vi "Main_Motor_Evaluation_Force.vi"(0 "VISA Refnum in":refnum<visa-resource-name>, 5 "Positions to reach":dbl[](array[numeric]), 11 "error in (no error)":errorcluster) -> (4 "VISA Refnum out":refnum<visa-resource-name>, 6 "Actual positions":dbl[](array[numeric]), 8 "Current (mA)":dbl[](array[numeric]), 15 "error out":errorcluster)   [LabVIEW 2015]
uses:
  <instrlib>/Dynamixel Motor/Dynamixel Motor.lvlib
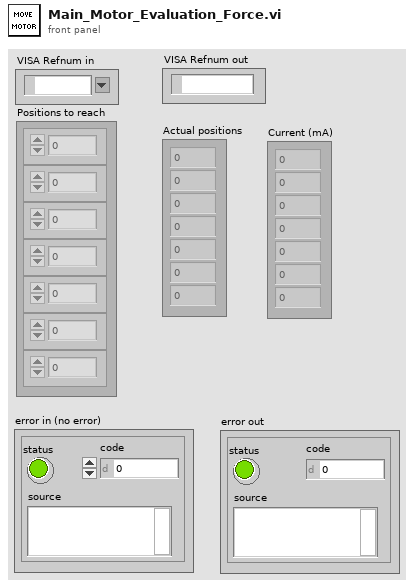
[diagram p1: front panel]
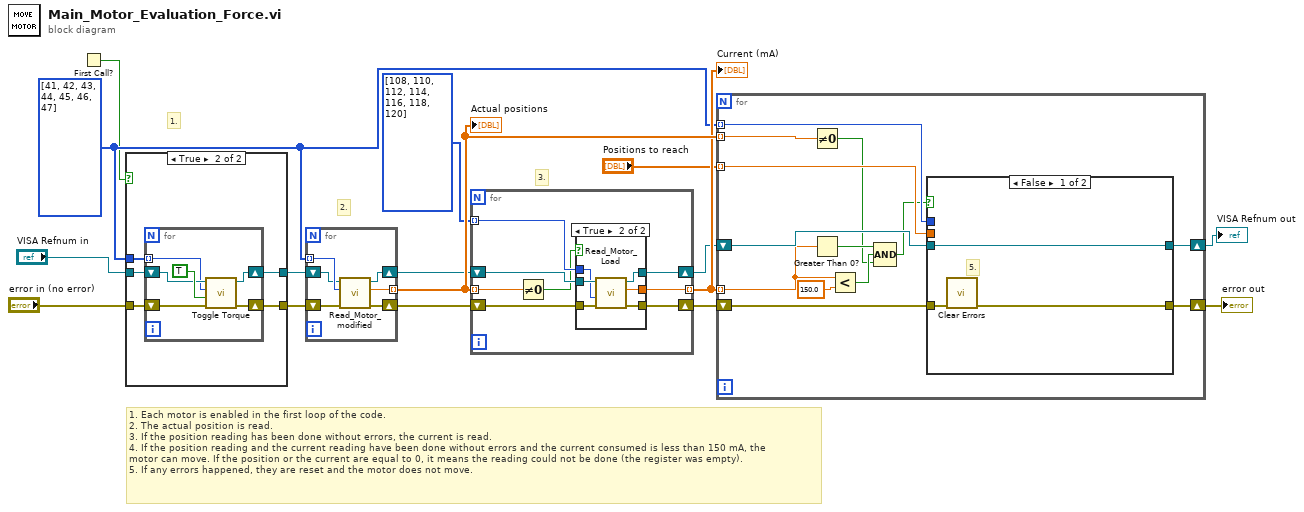
[diagram p0: block diagram]
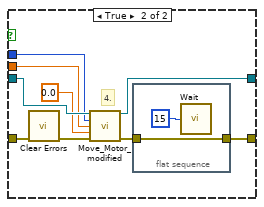
[diagram p2: hidden frame]
diagram:
  w6 = i32[] [41, 42, 43, 44, 45, 46, 47] ("y")
  # "3."
  # "2."
  # "1."
  # "1. Each motor is enabled in the first loop of the code.\n2. The actual position is read.\n3. If the position reading has been done without errors, the current is read.\n4. If the position reading and the current reading have been done without errors and the current consumed is less than 150 mA, the \nmotor can move. If the position or the current are equal to 0, it means the reading could not be done (the register was empty).\n5. If any errors happened, they are reset and the motor does not move."
  n1 = First Call?() -> (First Call?: T/F=w5:bool)
  n2 = case shown="True" w5 {
    tunnel: "VISA Refnum in" -> [w17 w23]
    tunnel: "error in (no error)" -> [w18 w22]
    tunnel: [w17 w21] -> w9
    tunnel: [w18 w20] -> w10
    tunnel: w6 -> [_ w19]
    frame False {
    }
    frame True {
      n3 = for {
        shift-right: [w27] -> w21
        shift-left: w23 -> [w28]
        shift-right: [w25] -> w20
        shift-left: w22 -> [w26]
        tunnel: w19 -> [w24] mode=indexing
        n4 = call <instrlib>:"Toggle Torque.vi"("error in (no error)"=w26, "Toggle torque (OFF)"=TRUE, "Motor ID (0)"=w24, "VISA resource name"=w28) -> ("error out"=w25:errorcluster, "VISA resource name out"=w27:refnum<visa-resource-name>)  [unwired: 6 in]
      }
    }
  }
  n5 = for {
    tunnel: w6 -> [w35] mode=indexing
    shift-right: [w30] -> w12
    shift-left: w10 -> [w34]
    shift-right: [w32] -> w11
    shift-left: w9 -> [w33]
    tunnel: [w31] -> w16 mode=indexing
    n6 = call "Read_Motor_modified.vi"("error in (no error)"=w34, "Motor ID (0)"=w35, "VISA Refnum in"=w33) -> ("error out"=w30:errorcluster, "Position"=w31:dbl, "VISA Refnum out"=w32:refnum<visa-resource-name>)  [unwired: 6 in]
  }
  "Actual positions" <- w16
  n7 = for {
    shift-right: [w42] -> w13
    shift-left: w11 -> [w43]
    shift-right: [w39] -> w14
    shift-left: w12 -> [w41]
    tunnel: [w38] -> w15 mode=indexing
    tunnel: u8[] [108, 110, 112, 114, 116, 118, 120] ("Address # DEC") -> [w40] mode=indexing
    tunnel: w16 -> [w37] mode=indexing
    n8 = Not Equal To 0?(x=w37) -> (x != 0?=w36:bool)
    n9 = case shown="True" w36 {
      tunnel: w43 -> [w45 w51]
      tunnel: [w45 w50] -> w42
      tunnel: w41 -> [w44 w49]
      tunnel: w40 -> [_ w48]
      tunnel: [w44 w46] -> w39
      tunnel: [_ w47] -> w38
      frame False {
      }
      frame True {
        n10 = call "Read_Motor_Load.vi"("error in (no error)"=w49, "Address"=w48, "VISA Refnum in"=w51) -> ("error out"=w46:errorcluster, "Current load"=w47:dbl, "VISA Refnum out"=w50:refnum<visa-resource-name>)  [unwired: 6 in]
      }
    }
  }
  "Current (mA)" <- w15
  n11 = for {
    shift-right: [w62] -> w1
    shift-left: w13 -> [w64]
    shift-right: [w59] -> w8
    shift-left: w14 -> [w63]
    tunnel: w6 -> [w61] mode=indexing
    tunnel: "Positions to reach" -> [w60] mode=indexing
    tunnel: w15 -> [w58] mode=indexing
    tunnel: w16 -> [w56] mode=indexing
    n12 = Not Equal To 0?(x=w56) -> (x != 0?=w53:bool)
    n13 = Greater Than 0?(x=w58) -> (x > 0?=w55:bool)
    n14 = Less?(x=w58, y=150.0) -> (x < y?=w54:bool)
    n15 = Compound Arithmetic op=AND(w55, w54, w53) -> (w52:bool)
    n16 = case shown="False" w52 {
      tunnel: w64 -> [w66 w76]
      tunnel: w63 -> [w67 w71]
      tunnel: [w66 w75] -> w62
      tunnel: w61 -> [_ w74]
      tunnel: w60 -> [_ w72]
      tunnel: [w65 w68] -> w59
      frame False {
        # "5."
        n17 = call <vilib>:"Clear Errors.vi"("error in (no error)"=w67) -> ("error out"=w65:errorcluster)  [unwired: 5 in, 1 out]
      }
      frame True {
        # "4."
        n18 = call <vilib>:"Clear Errors.vi"("error in (no error)"=w71) -> ("error out"=w70:errorcluster)  [unwired: 5 in, 1 out]
        n19 = call "Move_Motor_modified.vi"("VISA Refnum in"=w76, "Motor ID (0)"=w74, "Goal Position (bit)"=w72, "Goal Speed (RPM)"=0.0, "error in (no error)"=w70) -> ("VISA Refnum out"=w75:refnum<visa-resource-name>, "error out"=w69:errorcluster)  [unwired: 9 in]
        n20 = flat-sequence {
          tunnel: [w77] -> w68
          tunnel: w69 -> [w77]
          frame #0 {
            n21 = call "Wait"("Count(mSec)"=u32 15) -> ()  [unwired: 1 out]
          }
        }
      }
    }
  }
  "error out" <- w8
  "VISA Refnum out" <- w1
